vi "Evaluate Expression.vi"(8 "error in (no error)":errorcluster) -> (0 "error out":errorcluster)   [LabVIEW 2020]
uses:
  G-Embedded-Python-Interpreter-Toolkit/Merge Call Library Errors.vi
  <vilib>/addons/_JKI Toolkits/Caraya/classes/Assert/Assert Not Error.vi
  <vilib>/addons/_JKI Toolkits/Caraya/classes/Assert/Assert Equal Value and Type_Variant.vi
  G-Embedded-Python-Interpreter-Toolkit/G-Embedded-Python-Interpreter-Toolkit.lvlib
  <vilib>/addons/_JKI Toolkits/Caraya/classes/Test/Test.lvclass
  <vilib>/addons/_JKI Toolkits/Caraya/classes/Assert/Assert.lvclass
panel:
  out "Value":i32
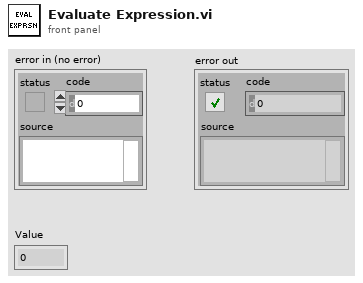
[diagram p1: front panel]
types:
  T1 = typedef "G-Embedded-Python-Interpreter-Toolkit.lvlib/Python Object Reference.ctl" = refnum<k1>
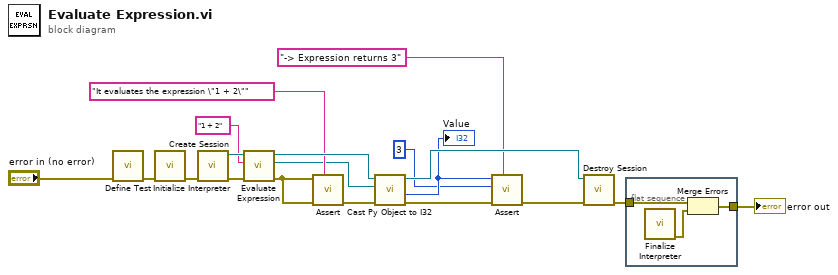
[diagram p0: block diagram]
diagram:
  n1 = call <vilib>:"Define Test.vi"("error in (no error)"="error in (no error)") -> ("error out"=w19:errorcluster)  [unwired: 10 in]
  n2 = call "Initialize Interpreter.vi"("error in (no error)"=w19) -> ("error out"=w16:errorcluster)  [unwired: 9 in, 1 out]
  n3 = call "Create Session.vi"("error in (no error)"=w16) -> ("error out"=w14:errorcluster, "Session Handle"=w15:refnum<data-value>)  [unwired: 9 in]
  n4 = call "Evaluate Expression.vi"("error in (no error)"=w14, "Expression"="1 + 2", "Session Handle in"=w15) -> ("error out"=w6:errorcluster, "Python Object Refnum"=w1:T1, "Session Handle out"=w12:refnum<data-value>)  [unwired: 6 in]
  n5 = call-poly <vilib>:"Assert.vi"("Label"="It evaluates the expression \"1 + 2\"", "error in (no error)"=w6, "Not Error?"=w6) -> ("error out"=w5:errorcluster)  [unwired: 8 in]
  n6 = call "Cast Py Object to I32.vi"("error in (no error)"=w5, "Python Object Refnum in"=w1, "Session Handle in"=w12) -> ("error out"=w4:errorcluster, "Value"=w10:i32, "Session Handle out"=w11:refnum<data-value>)  [unwired: 5 in, 1 out]
  "Value" <- w10
  n7 = call-poly <vilib>:"Assert.vi"("Label"="-> Expression returns 3", "error in (no error)"=w4, "Y"=3 ("Value"), "X"=w10) -> ("error out"=w9:errorcluster)  [unwired: 7 in]
  n8 = call "Destroy Session.vi"("error in (no error)"=w9, "Session Handle"=w11) -> ("error out"=w13:errorcluster)  [unwired: 9 in]
  n9 = flat-sequence {
    tunnel: w13 -> [w22]
    tunnel: [w20] -> w17
    frame #0 {
      n10 = call "Finalize Interpreter.vi"() -> ("error out"=w21:errorcluster)  [unwired: 11 in]
      n11 = Merge Errors(w22, w21) -> (w20:errorcluster)
    }
  }
  "error out" <- w17
